vi "AlliGator Create Max & Sum Images.vi"(5 "Prefix":string, 6 "Image Characteristics":T2 {"Calibration"."Y Step" format="%.2f"; "Calibration"."X Step" format="%.2f"; "Image Type" items=["Grayscale (U8)", "Grayscale (I16)", "Grayscale (SGL)", "Complex (CSG)", "RGB (U32)", "HSL (U32)", "RGB (U64)", "Grayscale (U16)"]}, 7 "Image Type":bool, 8 "Error In":errorcluster, 9 "Image Min":T1, 10 "Image Max":T1, 11 "Image Sum":T1) -> (0 "Error Out":errorcluster, 1 "Image Min":T1, 2 "Image Max":T1, 3 "Image Sum":T1)   [LabVIEW 2021, in "AlliGator Files.lvlib"]
doc: "Creates image structures for Sum, Min and Max images"
uses:
  AlliGator Files.lvlib
  <vilib>/vision/Image Controls.llb/IMAQ Image.ctl
  Image/Image Characteristics.ctl
  Image/Image.lvlib
panel:
  # "see the AlliGator License on the block diagram (Ctrl+E or Window:Show Block Diagram)"
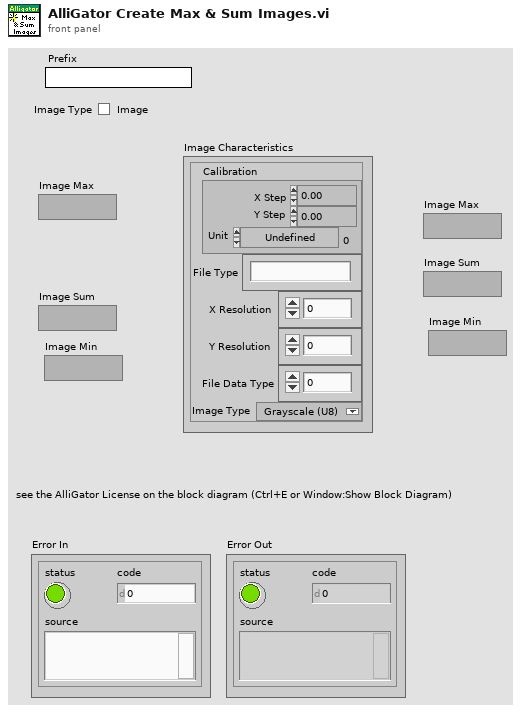
[diagram p1: front panel]
types:
  T1 = typedef "IMAQ Image.ctl" = refnum<image>
  T2 = typedef "Image.lvlib/Image Characteristics.ctl" = cluster{"Calibration":T3, "File Type":string, "X Resolution":i32, "Y Resolution":i32, "File Data Type":i32, "Image Type":T5}
  T3 = typedef "Simple Grid Descriptor" = cluster{"X Step":sgl, "Y Step":sgl, "Unit":T4}
  T4 = typedef "Image Unit" = enum32{"Undefined", "Angström", "Micrometer", "Millimeter", "Centimeter", "Meter", "Kilometer", "Microinch", "Inch", "Feet", "Nautical miles", "Standard miles", "Steps"}
  T5 = typedef "Image Type" = u32
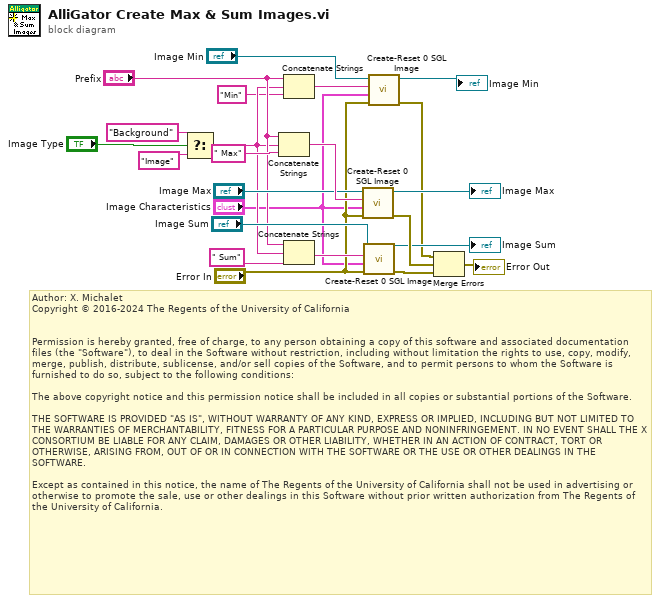
[diagram p0: block diagram]
diagram:
  # "Author: X. Michalet\nCopyright © 2016-2024 The Regents of the University of California\n \n\nPermission is hereby granted, free of charge, to any person obtaining a copy of this software and associated documentation files (the \"Software\"), to deal in the Software without restriction, including without limitation the rights to use, copy, modify, merge, publish, distribute, sublicense, and/or sell copies of the Software, and to permit persons to whom the Software is furnished to do so, subject to the following conditions:\n\nThe above copyright notice and this permission notice shall be included in all copies or substantial portions of the Software.\n\nTHE SOFTWARE IS PROVIDED \"AS IS\", WITHOUT WARRANTY OF ANY KIND, EXPRESS OR IMPLIED, INCLUDING BUT NOT LIMITED TO THE WARRANTIES OF MERCHANTABILITY, FITNESS FOR A PARTICULAR PURPOSE AND NONINFRINGEMENT. IN NO EVENT SHALL THE X CONSORTIUM BE LIABLE FOR ANY CLAIM, DAMAGES OR OTHER LIABILITY, WHETHER IN AN ACTION OF CONTRACT, TORT OR OTHERWISE, ARISING FROM, OUT OF OR IN CONNECTION WITH THE SOFTWARE OR THE USE OR OTHER DEALINGS IN THE SOFTWARE.\n\nExcept as contained in this notice, the name of The Regents of the University of California shall not be used in advertising or otherwise to promote the sale, use or other dealings in this Software without prior written authorization from The Regents of the University of California."
  n1 = Select(t="Background" ("x"), s="Image Type", f="Image") -> (s? t:f=w8:string)
  n2 = Concatenate Strings("Prefix", w8, " Max" ("Image Name")) -> (w21:string)
  n3 = Concatenate Strings("Prefix", w8, "Min" ("string")) -> (w6:string)
  n4 = Concatenate Strings("Prefix", w8, " Sum" ("Image Name")) -> (w22:string)
  n5 = call "Create-Reset 0 SGL Image.vi"("Error In"="Error In", "Image Characteristics"="Image Characteristics", "Image Name"=w21, "Image"="Image Max") -> ("Error Out"=w19:errorcluster, "New Image"=→"Image Max":T1)  [unwired: 6 in]
  n6 = call "Create-Reset 0 SGL Image.vi"("Error In"="Error In", "Image Characteristics"="Image Characteristics", "Image Name"=w22, "Image"="Image Sum") -> ("Error Out"=w18:errorcluster, "New Image"=→"Image Sum":T1)  [unwired: 6 in]
  n7 = call "Create-Reset 0 SGL Image.vi"("Error In"="Error In", "Image Characteristics"="Image Characteristics", "Image Name"=w6, "Image"="Image Min") -> ("Error Out"=w4:errorcluster, "New Image"=→"Image Min":T1)  [unwired: 6 in]
  n8 = Merge Errors(w4, w19, w18) -> (→"Error Out":errorcluster)
